vi "2_Analog_Meter_Reader(Training).vi"() -> ()   [LabVIEW 2020]
doc: "This example demonstrating the usage of Deep Learning toolkit for solving geometrical objects recognition problem based on Multilayer perceptron (MLP) and Convolutional Neural Network (CNN)."
uses:
  <vilib>/Ngene/DeepLTK/Toolkit/NN_Train/Controls/NN_LR_Policy_Cfg.ctl
  <vilib>/Ngene/DeepLTK/Toolkit/NN_Train/Controls/NN_LR_Policy_Type.ctl
  <vilib>/Ngene/DeepLTK/Toolkit/NN_Train/Controls/NN_Train_Params.ctl
  <vilib>/Ngene/DeepLTK/Toolkit/NN_Train/Controls/NN_Train_Optimizer.ctl
  <vilib>/Ngene/DeepLTK/Toolkit/NN_Train/Controls/NN_Train_Data_Sampling.ctl
  Controls/Regression_Report.ctl
  <vilib>/Ngene/DeepLTK/Toolkit/NN_Layers/Layers/FC/Controls/NN_Layer_Config(FC).ctl
  <vilib>/Ngene/DeepLTK/Toolkit/NN_Activations/Controls/NN_Activation_Type.ctl
  <vilib>/Ngene/DeepLTK/Toolkit/NN_Layers/Controls/NN_Layer_Init_Params.ctl
  <vilib>/Ngene/DeepLTK/Toolkit/NN_Layers/Controls/NN_Layer_Weight_Init_Type.ctl
  <vilib>/Ngene/DeepLTK/Toolkit/NN_Layers/Layers/Input/Controls/NN_Layer_Config(Input3D).ctl
  <vilib>/Ngene/DeepLTK/Toolkit/NN_Data/Controls/NN_Dims(C,H,W).ctl
  <vilib>/Ngene/DeepLTK/Toolkit/NN_Network/Controls/NN_Save_Before_Destroy_Options.ctl
  <vilib>/Ngene/DeepLTK/Toolkit/NN_Layers/Layers/Conv2D/Controls/NN_Layer_Config(Conv2D).ctl
  <vilib>/Ngene/DeepLTK/Toolkit/NN_Layers/Layers/Conv2D/Controls/NN_Layer_Params(Conv2D).ctl
  <vilib>/Ngene/DeepLTK/Toolkit/NN_Layers/Layers/Conv2D/Controls/NN_Conv2D_Padding_Type.ctl
  <vilib>/Ngene/DeepLTK/Toolkit/NN_Layers/Layers/DropOut3D/Controls/NN_Layer_Config(DropOut3D).ctl
  cd255efe-81e1-4e35-9bfd-5e2bf705b7ac.vi
  <vilib>/Ngene/DeepLTK/Toolkit/NN_Layers/Layers/Input/NN_Layer_Create(Input3D).vi
  <vilib>/Ngene/DeepLTK/Toolkit/NN_Layers/Layers/Conv2D/NN_Layer_Create(Conv2D).vi
  <vilib>/Ngene/DeepLTK/Toolkit/NN_Layers/Layers/DropOut3D/NN_Layer_Create(DropOut3D).vi
  <vilib>/Ngene/DeepLTK/Toolkit/NN_Layers/Layers/FC/NN_Layer_Create(FC).vi
  <vilib>/Ngene/DeepLTK/Toolkit/NN_Train/Loss_Functions/NN_Set_Loss(MSE).vi
  <vilib>/ptbypt/Filters.llb/FIR Filter PtByPt.vi
  <vilib>/Ngene/DeepLTK/Toolkit/NN_Network/subVIs/NN_Predict/NN_Predict(In3D_Out1D).vi
  <vilib>/Ngene/DeepLTK/Toolkit/NN_Train/Eval_Loss/NN_Eval_Test_Error_Loss/NN_Eval(In3D_Out1D).vi
  <vilib>/Ngene/DeepLTK/Toolkit/NN_Data/subVIs/Dataset_Destroy/NN_Datasets_All_Destroy(In3D_Out1D).vi
  <vilib>/Ngene/DeepLTK/Toolkit/Deep_Learning_Toolkit_by_Ngene.lvlib
panel:
  in  "NN Device":enum16{"CPU", "GPU"}(ring)=enum."GPU"
  out "Train Speed (img/s)":dbl=1665.0883017080685 format="%#_3p"
  out "Train Speed (sec/batch)":dbl=0.07687280000027386 format="%#_3p"
  out "Elapsed Time":dbl=38.292933199998515 format="%<%H:%M:%S>t"
  out "Test.Dataset_Size":i32=200
  out "Train.Dataset_Size":i32=1000
  out "Loss Values":cluster{"Train_Loss":dbl, "Test_Loss":dbl}={"Train_Loss"=19.829761505126953, "Test_Loss"=0.26563704013824463} {"Test_Loss" format="%#_4g"}
  out "Session Data":T1={"Epochs"=60.03200149536133, "Tot_Iter"=469.0, "LR"=0.625, "LR_iter"=470.0} {"LR" format="%#_3g"}
  out "Loss Charts":cluster{"Filtered x":sgl, "Test_Loss":sgl}(graph)={"Filtered x"=19.829762, "Test_Loss"=0.26563704}
  in  "Image Folder(Test)":path=path "D:/DeepLTK_Examples/Analog_Meter/Test/Images"
  in  "Labels (Test)":path=path "D:/DeepLTK_Examples/Analog_Meter/Test/Labels.csv"
  in  "Stop":bool
  out "Regression Metrics":T2={"Graphs"=[{"Best Linear Fit"=[0.0, 0.7035179734230042, 1.407034993171692, 2.110553026199341, 2.814069986343384, 3.517587900161743, 4.221106052398682, 4.924623012542725, 5.628140926361084, 6.331657886505127, 7.035175800323486, 7.7386932373046875, 8.442211151123047, 9.145729064941406, 9.84924602508545, 10.552763938903809, 11.256280899047852, 11.959798812866211, 12.66331672668457, 13.366833686828613, 14.070351600646973, 14.773868560791016, 15.477387428283691, 16.180904388427734, 16.884422302246094, 17.587940216064453, 18.29145622253418, 18.99497413635254, 19.6984920501709, 20.402009963989258, 21.105527877807617, 21.809045791625977, 22.512563705444336, 23.216079711914062, 23.919597625732422, 24.62311553955078, 25.32663345336914, 26.0301513671875, 26.733667373657227, 27.437185287475586, 28.140703201293945, 28.844221115112305, 29.547739028930664, 30.251256942749023, 30.954774856567383, 31.65829086303711, 32.36180877685547, 33.06532669067383, 33.76884460449219, 34.47236251831055, 35.175880432128906, 35.879398345947266, 36.582916259765625, 37.28643035888672, 37.98994827270508, 38.69346618652344, 39.3969841003418, 40.100502014160156, 40.804019927978516, 41.507537841796875, 42.211055755615234, 42.914573669433594, 43.61809158325195, 44.32160949707031, 45.02512741088867, 45.728641510009766, 46.432159423828125, 47.135677337646484, 47.839195251464844, 48.5427131652832, 49.24623107910156, 49.94974899291992, 50.65326690673828, 51.35678482055664, 52.060302734375, 52.76382064819336, 53.46733856201172, 54.17085266113281, 54.87437057495117, 55.57788848876953, 56.28140640258789, 56.98492431640625, 57.68844223022461, 58.39196014404297, 59.09547805786133, 59.79899597167969, 60.50251388549805, 61.206031799316406, 61.909549713134766, 62.61306381225586, 63.31658172607422, 64.02010345458984, 64.72361755371094, 65.42713928222656, 66.13065338134766, 66.83416748046875, 67.53768920898438, 68.24120330810547, 68.9447250366211, 69.64823913574219, 70.35176086425781, 71.0552749633789, 71.75879669189453, 72.46231079101562, 73.16583251953125, 73.86934661865234, 74.57286071777344, 75.27638244628906, 75.97989654541016, 76.68341827392578, 77.38693237304688, 78.0904541015625, 78.7939682006836, 79.49748992919922, 80.20100402832031, 80.90452575683594, 81.60803985595703, 82.31156158447266, 83.01507568359375, 83.71858978271484, 84.42211151123047, 85.12562561035156, 85.82914733886719, 86.53266143798828, 87.2361831665039, 87.939697265625, 88.64321899414062, 89.34673309326172, 90.05024719238281, 90.75376892089844, 91.45728302001953, 92.16080474853516, 92.86431884765625, 93.56784057617188, 94.27135467529297, 94.9748764038086, 95.67839050292969, 96.38191223144531, 97.0854263305664, 97.78894805908203, 98.49246215820312, 99.19597625732422, 99.89949798583984, 100.60301208496094, 101.30653381347656, 102.01004791259766, 102.71356964111328, 103.41708374023438, 104.12060546875, 104.8241195678711, 105.52764129638672, 106.23115539550781, 106.9346694946289, 107.63819122314453, 108.34170532226562, 109.04522705078125, 109.74874114990234, 110.45226287841797, 111.15577697753906, 111.85929870605469, 112.56281280517578, 113.2663345336914, 113.9698486328125, 114.67337036132812, 115.37688446044922, 116.08039855957031, 116.78392028808594, 117.48743438720703, 118.19095611572266, 118.89447021484375, 119.59799194335938, 120.30150604248047, 121.0050277709961, 121.70854187011719, 122.41206359863281, 123.1155776977539, 123.819091796875, 124.52261352539062, 125.22612762451172, 125.92964935302734, 126.63316345214844, 127.33668518066406, 128.0402069091797, 128.74371337890625, 129.44723510742188, 130.1507568359375, 130.85427856445312, 131.5577850341797, 132.2613067626953, 132.96482849121094, 133.6683349609375, 134.37185668945312, 135.07537841796875, 135.77890014648438, 136.48240661621094, 137.18592834472656, 137.8894500732422, 138.5929718017578, 139.29647827148438, 140.0], "Array 3"=[1.2962517, 0.8418449, 2.5273826, 2.343565, 2.8205507, 3.8072836, 4.6100063, 5.491647, 5.592317, 6.4402056, 7.130179, 7.626676, 8.663867, 9.402606, 10.082472, 10.911277, 11.306467, 11.893557, 12.946919, 13.433682, 14.082973, 14.6786, 15.393217, 16.218815, 16.990051, 17.676376, 18.30693, 19.016312, 19.612173, 20.773912, 21.31578, 22.13029, 22.531034, 23.691423, 23.968306, 24.432058, 25.35231, 25.968063, 26.499355, 27.619349, 28.226751, 28.762365, 29.584696, 30.380968, 30.965748, 31.767052, 32.254795, 32.90442, 33.4425, 33.98359, 35.325848, 36.042965, 36.61501, 37.261543, 37.82164, 38.58534, 39.109116, 39.722027, 40.41493, 40.994183, 41.832478, 42.44226, 43.27765, 44.356384, 44.996952, 45.652363, 46.350983, 46.879814, 47.487907, 48.07724, 48.716225, 49.195232, 50.24242, 51.0404, 51.87234, 52.24179, 52.91254, 53.425343, 54.369644, 55.455452, 56.149426, 56.705288, 57.2974, 57.85313, 58.777023, 59.593285, 60.04869, 60.95353, 61.77137, 62.53276, 63.122807, 63.74631, 64.20286, 65.17948, 65.843544, 66.83675, 67.39386, 68.15095, 68.68514, 69.15952, 69.499016, 70.364685, 71.12549, 72.3465, 72.72487, 73.790794, 74.30419, 74.74704, 75.398346, 76.282745, 77.012344, 77.77125, 78.58103, 79.15686, 79.749214, 80.42085, 81.20427, 81.76548, 82.57208, 83.061516, 83.735374, 84.47109, 85.10138, 85.91469, 86.56425, 87.1886, 88.19484, 88.94755, 89.88243, 90.78077, 91.201805, 92.01801, 92.4638, 92.76064, 93.48943, 94.34645, 95.05727, 95.58946, 96.37274, 96.85058, 97.76942, 98.29599, 99.13515, 99.81821, 100.50452, 101.524635, 102.11071, 102.60852, 103.29312, 103.88792, 104.80595, 105.36168, 106.023285, 106.71556, 107.36465, 108.053665, 108.94084, 109.85283, 110.555466, 111.16668, 111.92209, 113.046684, 113.679955, 114.0655, 115.12781, 115.78996, 116.65573, 116.89387, 117.78699, 118.39015, 119.00426, 120.01063, 120.73522, 121.56977, 122.11879, 122.91684, 123.60596, 124.266556, 125.044495, 125.64256, 126.34403, 126.98127, 127.77769, 128.66357, 128.89668, 129.37943, 130.17139, 130.81459, 131.21861, 132.22198, 133.08286, 133.59778, 134.10455, 134.84381, 135.72055, 137.03716, 137.40094, 137.66003, 137.51796, 138.29012]}, {"Best Linear Fit"=[1.1465655086328974, 0.6890048561897085, 2.3862414129443907, 2.201147959522832, 2.6814442810750747, 3.6750258871861514, 4.48332006058631, 5.371079722444516, 5.472448785683747, 6.326222219723485, 7.020984492338908, 7.520927698919899, 8.56531747444022, 9.309183875628419, 9.993768477460348, 10.828325958184701, 11.226259105607417, 11.817423473743009, 12.87809742648757, 13.368238917194887, 14.022035548748985, 14.621797424694607, 15.341374161798484, 16.17270217544307, 16.949291538335128, 17.640380208121634, 18.275310913345354, 18.98961563907013, 19.589612786926114, 20.759415454631, 21.305044625029957, 22.125206345720784, 22.52873320284901, 23.697176094941362, 23.97598003077316, 24.442951559630774, 25.369590624896187, 25.989617574818702, 26.524597090173177, 27.652363869697975, 28.26398248963226, 28.803314055181648, 29.631352103255235, 30.433151091415798, 31.021989628666113, 31.828855125394277, 32.319983797831604, 32.974116532114785, 33.51593333727239, 34.0607769875788, 35.412351693521735, 36.13444632021322, 36.71046109790862, 37.361482481213976, 37.9254667017951, 38.69446590477087, 39.22187830725335, 39.83904358251107, 40.53675443635409, 41.12002903299775, 41.96414239445679, 42.57815790699621, 43.419344293831664, 44.505566855454354, 45.150580642550665, 45.8105404378627, 46.514009211601724, 47.04651116969608, 47.65882504213281, 48.252248020607865, 48.8956677204748, 49.37800010434517, 50.43245615660163, 51.23597599073511, 52.07368995623235, 52.44570382148143, 53.12110897763525, 53.63747032238536, 54.588326069428206, 55.681670167733486, 56.38046039148363, 56.94018090887292, 57.536404103228016, 58.095990179525664, 59.02629564541866, 59.848222385583945, 60.306789425627365, 61.21790822715708, 62.0414252133777, 62.80810050605522, 63.402241784077006, 64.03007399966242, 64.48978955074581, 65.47319156548636, 66.14186314353631, 67.14195890068385, 67.70293932316045, 68.46528177151329, 69.0031844203173, 69.48085746006902, 69.82270658552935, 70.69438421194752, 71.46046796382186, 72.68995095269035, 73.07094932403467, 74.14427322320853, 74.66123379110992, 75.1071556861916, 75.76298237822938, 76.65352016921686, 77.38818311738916, 78.15235396458823, 78.96775839122222, 79.54758361357194, 80.14404880189198, 80.82034895159869, 81.60920318322187, 82.17430902662463, 82.98650991410366, 83.47934022664367, 84.15787593964555, 84.89870013098877, 85.53336195402922, 86.35231562548235, 87.00638305980674, 87.63506801603052, 88.64829290606968, 89.4062256866169, 90.34759757493845, 91.25217101589257, 91.67612907777522, 92.49800204150384, 92.94688164060149, 93.24578644021967, 93.97963505949407, 94.84260090317433, 95.55834991034067, 96.0942397839442, 96.8829557333017, 97.36410887673973, 98.28932478702085, 98.81955277007955, 99.66453423687315, 100.35233486167569, 101.043408166766, 102.07060724798706, 102.66074986382623, 103.1620153945728, 103.85136785369019, 104.45029139340012, 105.37469297478334, 105.93428289225504, 106.6004807542189, 107.29756165551828, 107.95115278426087, 108.64495332292435, 109.53828748861784, 110.45660465031106, 111.16411818032128, 111.77957413312821, 112.5402264649005, 113.67262762091265, 114.31029324205761, 114.69851302060974, 115.76819548678732, 116.43494647781392, 117.30672397475732, 117.54651310579675, 118.445831820655, 119.05318289622339, 119.67155045895774, 120.68490594891448, 121.4145292767375, 122.25487060528268, 122.80770005643218, 123.6112890316985, 124.3051894408872, 124.97037323290274, 125.75371153859486, 126.35593080563686, 127.06226893638878, 127.70392937854231, 128.50587433131665, 129.39791018018235, 129.63263664382822, 130.11872953709033, 130.91618799857812, 131.5638560369407, 131.97068246257504, 132.98101878973108, 133.8478642191985, 134.36636125671856, 134.8766535464749, 135.62104234733346, 136.50386706083515, 137.829609871314, 138.19591959310375, 138.45681213435577, 138.3137514481604, 139.0912665339977], "Array 3"=[1.2962517, 0.8418449, 2.5273826, 2.343565, 2.8205507, 3.8072836, 4.6100063, 5.491647, 5.592317, 6.4402056, 7.130179, 7.626676, 8.663867, 9.402606, 10.082472, 10.911277, 11.306467, 11.893557, 12.946919, 13.433682, 14.082973, 14.6786, 15.393217, 16.218815, 16.990051, 17.676376, 18.30693, 19.016312, 19.612173, 20.773912, 21.31578, 22.13029, 22.531034, 23.691423, 23.968306, 24.432058, 25.35231, 25.968063, 26.499355, 27.619349, 28.226751, 28.762365, 29.584696, 30.380968, 30.965748, 31.767052, 32.254795, 32.90442, 33.4425, 33.98359, 35.325848, 36.042965, 36.61501, 37.261543, 37.82164, 38.58534, 39.109116, 39.722027, 40.41493, 40.994183, 41.832478, 42.44226, 43.27765, 44.356384, 44.996952, 45.652363, 46.350983, 46.879814, 47.487907, 48.07724, 48.716225, 49.195232, 50.24242, 51.0404, 51.87234, 52.24179, 52.91254, 53.425343, 54.369644, 55.455452, 56.149426, 56.705288, 57.2974, 57.85313, 58.777023, 59.593285, 60.04869, 60.95353, 61.77137, 62.53276, 63.122807, 63.74631, 64.20286, 65.17948, 65.843544, 66.83675, 67.39386, 68.15095, 68.68514, 69.15952, 69.499016, 70.364685, 71.12549, 72.3465, 72.72487, 73.790794, 74.30419, 74.74704, 75.398346, 76.282745, 77.012344, 77.77125, 78.58103, 79.15686, 79.749214, 80.42085, 81.20427, 81.76548, 82.57208, 83.061516, 83.735374, 84.47109, 85.10138, 85.91469, 86.56425, 87.1886, 88.19484, 88.94755, 89.88243, 90.78077, 91.201805, 92.01801, 92.4638, 92.76064, 93.48943, 94.34645, 95.05727, 95.58946, 96.37274, 96.85058, 97.76942, 98.29599, 99.13515, 99.81821, 100.50452, 101.524635, 102.11071, 102.60852, 103.29312, 103.88792, 104.80595, 105.36168, 106.023285, 106.71556, 107.36465, 108.053665, 108.94084, 109.85283, 110.555466, 111.16668, 111.92209, 113.046684, 113.679955, 114.0655, 115.12781, 115.78996, 116.65573, 116.89387, 117.78699, 118.39015, 119.00426, 120.01063, 120.73522, 121.56977, 122.11879, 122.91684, 123.60596, 124.266556, 125.044495, 125.64256, 126.34403, 126.98127, 127.77769, 128.66357, 128.89668, 129.37943, 130.17139, 130.81459, 131.21861, 132.22198, 133.08286, 133.59778, 134.10455, 134.84381, 135.72055, 137.03716, 137.40094, 137.66003, 137.51796, 138.29012]}, {"Best Linear Fit"=[0.0, 140.0], "Array 3"=[0.0, 140.0]}], "y=k*x+b"="y = 0.993*x + 0.158", "R"=0.9999755, "R^2"=0.999951, "MAE"=0.40923384, "MSE"=0.26563704} {"R" format="%#_7g"}
  in  "Evaluate Model":bool
  in  "LR Update Policy":T3={"Policy_Type"=enum."Step", "LR0"=20.0, "k"=10.0, "WarmUp_Policy"=enum."Ramp", "WarmUp_Iter"=50, "WarmUp_Ratio"=50.0} {"WarmUp_Ratio" min=1; "WarmUp_Iter" min=1; "LR0" format="%.7f"}
  in  "Train_Params":T5={"Optimizer"=enum."Adam", "Beta_1"=0.9, "Beta_2"=0.999, "Weight Decay(L1)"=3e-09, "Weight Decay(L2)"=3e-09, "Data_Sampling"=enum."Random"}
  in  "Image Folder(Train)":path=path "D:/DeepLTK_Examples/Analog_Meter/Train/Images"
  in  "Labels (Train)":path=path "D:/DeepLTK_Examples/Analog_Meter/Train/Labels.csv"
  in  "Max_Epochs_to_Train":sgl=60.0
  in  "Input Height":i32=256
  in  "Input Width":i32=256
  out "Test_Loss":sgl=0.26563704
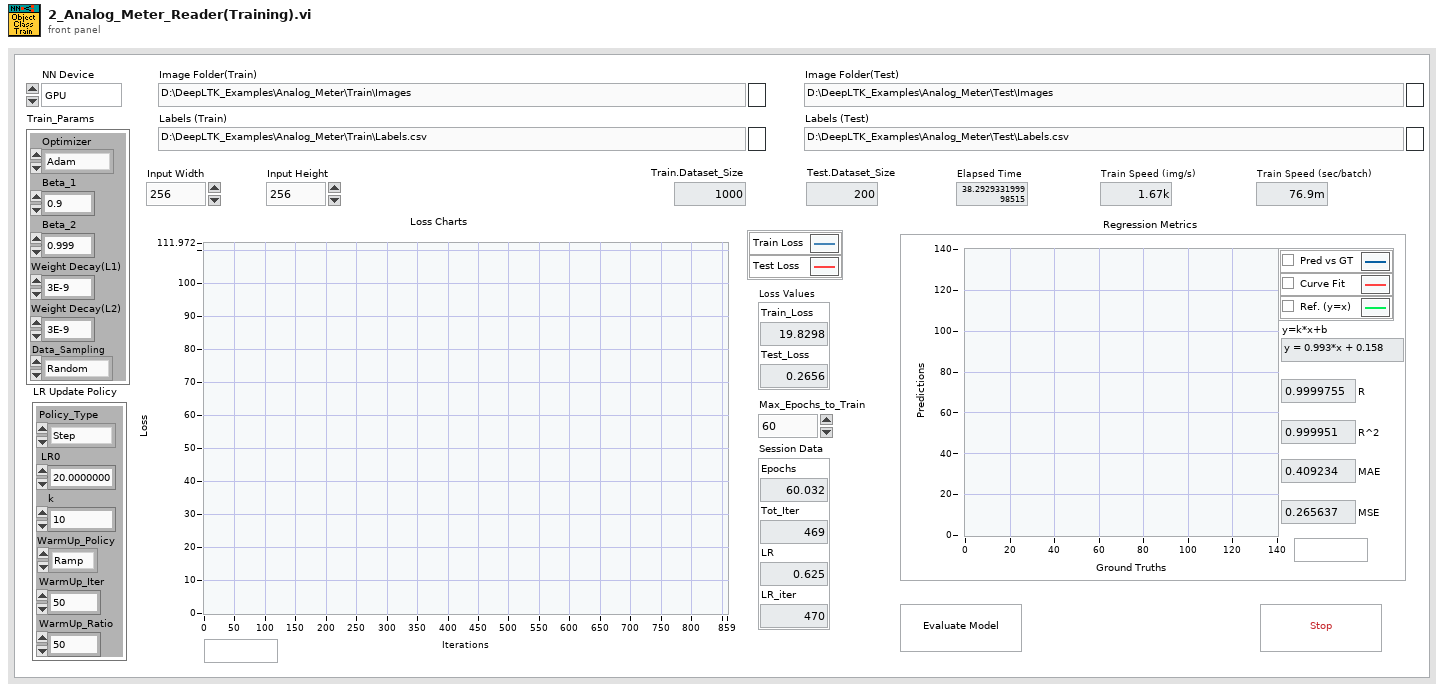
[diagram p1: front panel]
types:
  T1 = cluster{"Epochs":dbl, "Tot_Iter":dbl, "LR":dbl, "LR_iter":dbl}
  T2 = typedef "Regression_Report.ctl" = cluster{"Graphs":cluster{"Best Linear Fit":dbl[], "Array 3":sgl[]}[], "y=k*x+b":string, "R":sgl, "R^2":sgl, "MAE":sgl, "MSE":sgl}
  T3 = typedef "Deep_Learning_Toolkit_by_Ngene.lvlib/NN_LR_Policy_Cfg.ctl" = cluster{"Policy_Type":T4, "LR0":dbl, "k":sgl, "WarmUp_Policy":enum16{"Step", "Ramp"}, "WarmUp_Iter":i32, "WarmUp_Ratio":sgl}
  T4 = typedef "Deep_Learning_Toolkit_by_Ngene.lvlib/NN_LR_Policy_Type.ctl" = enum16{"Manual", "Step", "Exp", "1/t"}
  T5 = typedef "Deep_Learning_Toolkit_by_Ngene.lvlib/NN_Train_Params.ctl" = cluster{"Optimizer":T6, "Beta_1":sgl, "Beta_2":sgl, "Weight Decay(L1)":sgl, "Weight Decay(L2)":sgl, "Data_Sampling":T7}
  T6 = typedef "Deep_Learning_Toolkit_by_Ngene.lvlib/NN_Train_Optimizer.ctl" = enum16{"SGD", "Adam", "Adagrad", "Adadelta", "RMSProp", "Nesterov"}
  T7 = typedef "Deep_Learning_Toolkit_by_Ngene.lvlib/NN_Train_Data_Sampling.ctl" = enum16{"Random", "Sequential"}
  T8 = typedef "Deep_Learning_Toolkit_by_Ngene.lvlib/NN_Layer_Config(DropOut3D).ctl" = cluster{"Name":string, "Probability":sgl}
  T9 = typedef "Deep_Learning_Toolkit_by_Ngene.lvlib/NN_Layer_Config(FC).ctl" = cluster{"Name":string, "Size":i32, "BN":bool, "Activation":T10, "Init_Params":T11, "Custom_Params":string}
  T10 = typedef "Deep_Learning_Toolkit_by_Ngene.lvlib/NN_Activation_Type.ctl" = enum16{"Sigmoid", "ReLU", "LReLU", "ReLU6", "tanh", "Swish", "Mish", "None"}
  T11 = typedef "Deep_Learning_Toolkit_by_Ngene.lvlib/NN_Layer_Init_Params.ctl" = cluster{"Init_Type":T12, "Value":sgl}
  T12 = typedef "Deep_Learning_Toolkit_by_Ngene.lvlib/NN_Layer_Weight_Init_Type.ctl" = enum16{"Const", "Uniform", "Gaussian", "Xavier"}
  T13 = typedef "Deep_Learning_Toolkit_by_Ngene.lvlib/NN_Layer_Config(Conv2D).ctl" = cluster{"Name":string, "Conv_Params":T14, "BN?":bool, "Activation":T10, "Init_Params":T11, "Custom_Params":string}
  T14 = typedef "Deep_Learning_Toolkit_by_Ngene.lvlib/NN_Layer_Params(Conv2D).ctl" = cluster{"Filters":i32, "Kernel_Size":i32, "Stride":i32, "Pad_Type":T15, "Pad_Size":i32}
  T15 = typedef "Deep_Learning_Toolkit_by_Ngene.lvlib/NN_Conv2D_Padding_Type.ctl" = enum16{"Pad_Size", "Valid", "Same"}
  T16 = typedef "Deep_Learning_Toolkit_by_Ngene.lvlib/NN_Save_Before_Destroy_Options.ctl" = cluster{"CFG?":bool, "Weights?":bool, "Render?":bool}
  T17 = typedef "Deep_Learning_Toolkit_by_Ngene.lvlib/NN_Layer_Config(Input3D).ctl" = cluster{"Name":string, "Dims":T18}
  T18 = typedef "Deep_Learning_Toolkit_by_Ngene.lvlib/NN_Dims(C,H,W).ctl" = cluster{"C":i32, "H":i32, "W":i32}
  T19 = typedef "Deep_Learning_Toolkit_by_Ngene.lvlib/NN_DataSets_All(In3D_Out1D).ctl" = cluster{"Train":T20, "Validation":T20, "Test":T20}
  T20 = typedef "Deep_Learning_Toolkit_by_Ngene.lvlib/NN_DataSet(In3D_Out1D).ctl" = cluster{"Inputs Ref.":T21, "Outputs Ref.":T22, "Dataset_Size":i32, "Outputs_idx Ref.":T23, "Dims_In":T18, "Dims_Out":i32, "Labels":string[], "File Paths":path[]}
  T21 = typedef "Deep_Learning_Toolkit_by_Ngene.lvlib/NN_Data_ref(4D_SGL).ctl" = refnum<data-value>
  T22 = typedef "Deep_Learning_Toolkit_by_Ngene.lvlib/NN_Data_ref(2D_SGL).ctl" = refnum<data-value>
  T23 = typedef "Deep_Learning_Toolkit_by_Ngene.lvlib/NN_Data_ref(1D_I32).ctl" = refnum<data-value>
  T24 = typedef "Deep_Learning_Toolkit_by_Ngene.lvlib/NN.ctl" = cluster{"Name":string, "No of Layers":i32, "mBatch":i32, "Layers":T25[], "Dimty":T26, "Dims_In":T18, "Dims_Out":T18, "Working_Dir":path, "Train?":bool, "Train_Params":T5, "LR_Update_Policy":T3, "Session Data":T27, "Ground_truth":T28, "NNg_hdls":T29, "NN_Device":T30, "GPU Id":i32, "Labels":string[], "Receptive Field":T31[], "Loss_Type":T32, "Loss_Cfg_Prms":variant}
  T25 = typedef "Deep_Learning_Toolkit_by_Ngene.lvlib/NN_Layer_ref.ctl" = refnum<data-value>
  T26 = typedef "Deep_Learning_Toolkit_by_Ngene.lvlib/NN_In_Out_Dim-ty.ctl" = enum8{"In1D_Out1D", "In3D_Out1D", "In3D_Out3D", "In3D_OutBBox"}
  T27 = typedef "Deep_Learning_Toolkit_by_Ngene.lvlib/NN_Train_Session_Data.ctl" = cluster{"Epochs":sgl, "Tot_Iter":i32, "LR":sgl, "LR_iter":i32}
  T28 = typedef "Deep_Learning_Toolkit_by_Ngene.lvlib/NN_Ground_truth.ctl" = cluster{"Y":variant, "Y_idx":T23}
  T29 = typedef "Deep_Learning_Toolkit_by_Ngene.lvlib/nng_cuda_handles.ctl" = cluster{"cudnn":u64, "cublas":u64, "stream":u64, "curand":u64}
  T30 = typedef "Deep_Learning_Toolkit_by_Ngene.lvlib/NN_Device.ctl" = enum16{"CPU", "GPU"}
  T31 = typedef "Deep_Learning_Toolkit_by_Ngene.lvlib/NN_Dims(V,H).ctl" = cluster{"V":i32, "H":i32}
  T32 = typedef "Deep_Learning_Toolkit_by_Ngene.lvlib/NN_Loss_Type.ctl" = enum16{"None", "MSE", "CrossEntropy", "YOLO_v2"}
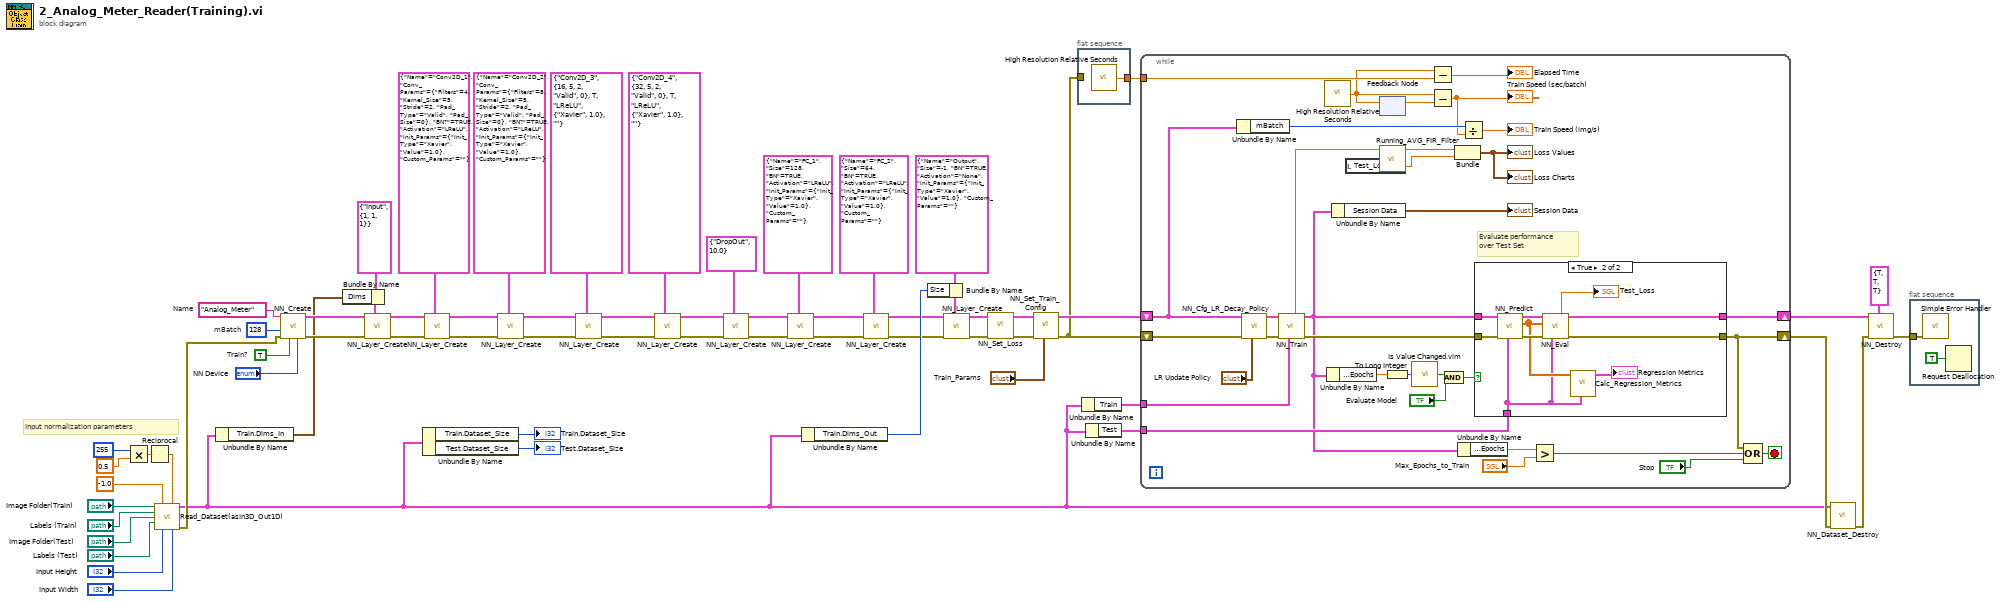
[diagram p0: block diagram]
diagram:
  w47 = TRUE  # Train?
  w59 = 128  # mBatch
  w64 = "Analog_Meter"  # Name
  # "Input normalization parameters"
  n1 = Multiply(x=u16 255 ("Shift"), y=sgl 0.5 ("Scale")) -> (x*y=w20:sgl)
  n2 = Reciprocal(x=w20) -> (1/x=w19:sgl)
  n3 = call "Read_Dataset(asIn3D_Out1D).vi"("Image Folder Path(Train)"="Image Folder(Train)", "Norm. Shift"=sgl -1.0 ("Scale"), "Norm. Scale"=w19, "Label File Path(Train)"="Labels (Train)", "Image Folder Path(Test)"="Image Folder(Test)", "Label File Path(Test)"="Labels (Test)", "Img Heigth"="Input Height", "Img Width"="Input Width") -> ("Datasets"=w1:T19, "error out"=w65:errorcluster)  [unwired: 6 in]
  n4 = Unbundle By Name(w1) -> ("Train.Dims_In"=w42:T18)
  n5 = call <vilib>:"NN_Create.vi"("NN_Device"="NN Device", "Train? (false)"=w47, "error in (no error)"=w65, "mBatch (1)"=w59, "Name"=w64) -> ("error out"=w62:errorcluster, "NN out"=w63:T24)  [unwired: 5 in]
  n6 = Bundle By Name(cluster=T17 {"Name"="Input", "Dims"={"C"=1, "H"=1, "W"=1}} ("Cluster"), "Dims"=w42) -> (w50:T17)
  n7 = call-poly <vilib>:"NN_Layer_Create.vi"("Input3D_Cfg"=w50, "error in (no error)"=w62, "NN In"=w63) -> ("error out"=w56:errorcluster, "NN out"=w57:T24)  [unwired: 6 in, 1 out]
  n8 = Unbundle By Name(w1) -> ("Train.Dataset_Size"=→"Train.Dataset_Size":i32, "Test.Dataset_Size"=→"Test.Dataset_Size":i32)
  n9 = call-poly <vilib>:"NN_Layer_Create.vi"("Conv2D_Cfg"=T13 {"Name"="Conv2D_1", "Conv_Params"={"Filters"=4, "Kernel_Size"=5, "Stride"=2, "Pad_Type"=enum."Valid", "Pad_Size"=0}, "BN?"=TRUE, "Activation"=enum."LReLU", "Init_Params"={"Init_Type"=enum."Xavier", "Value"=1.0}, "Custom_Params"=""}, "error in (no error)"=w56, "NN in"=w57) -> ("error out"=w16:errorcluster, "NN out"=w15:T24)  [unwired: 6 in, 1 out]
  n10 = call-poly <vilib>:"NN_Layer_Create.vi"("Conv2D_Cfg"=T13 {"Name"="Conv2D_2", "Conv_Params"={"Filters"=8, "Kernel_Size"=5, "Stride"=2, "Pad_Type"=enum."Valid", "Pad_Size"=0}, "BN?"=TRUE, "Activation"=enum."LReLU", "Init_Params"={"Init_Type"=enum."Xavier", "Value"=1.0}, "Custom_Params"=""}, "error in (no error)"=w16, "NN in"=w15) -> ("error out"=w39:errorcluster, "NN out"=w40:T24)  [unwired: 6 in, 1 out]
  n11 = call-poly <vilib>:"NN_Layer_Create.vi"("Conv2D_Cfg"=T13 {"Name"="Conv2D_3", "Conv_Params"={"Filters"=16, "Kernel_Size"=5, "Stride"=2, "Pad_Type"=enum."Valid", "Pad_Size"=0}, "BN?"=TRUE, "Activation"=enum."LReLU", "Init_Params"={"Init_Type"=enum."Xavier", "Value"=1.0}, "Custom_Params"=""}, "error in (no error)"=w39, "NN in"=w40) -> ("error out"=w7:errorcluster, "NN out"=w8:T24)  [unwired: 6 in, 1 out]
  n12 = call-poly <vilib>:"NN_Layer_Create.vi"("Conv2D_Cfg"=T13 {"Name"="Conv2D_4", "Conv_Params"={"Filters"=32, "Kernel_Size"=5, "Stride"=2, "Pad_Type"=enum."Valid", "Pad_Size"=0}, "BN?"=TRUE, "Activation"=enum."LReLU", "Init_Params"={"Init_Type"=enum."Xavier", "Value"=1.0}, "Custom_Params"=""}, "error in (no error)"=w7, "NN in"=w8) -> ("error out"=w5:errorcluster, "NN out"=w6:T24)  [unwired: 6 in, 1 out]
  n13 = call-poly <vilib>:"NN_Layer_Create.vi"("DropOut3D_Cfg"=T8 {"Name"="DropOut", "Probability"=10.0}, "error in (no error)"=w5, "NN in"=w6) -> ("error out"=w3:errorcluster, "NN out"=w4:T24)  [unwired: 6 in, 1 out]
  n14 = call-poly <vilib>:"NN_Layer_Create.vi"("FC_Cfg"=T9 {"Name"="FC_1", "Size"=128, "BN"=TRUE, "Activation"=enum."LReLU", "Init_Params"={"Init_Type"=enum."Xavier", "Value"=1.0}, "Custom_Params"=""} ("Layer_Config_Params"), "error in (no error)"=w3, "NN in"=w4) -> ("error out"=w17:errorcluster, "NN out"=w18:T24)  [unwired: 6 in, 1 out]
  n15 = Unbundle By Name(w1) -> ("Train.Dims_Out"=w41:i32)
  n16 = call-poly <vilib>:"NN_Layer_Create.vi"("FC_Cfg"=T9 {"Name"="FC_2", "Size"=64, "BN"=TRUE, "Activation"=enum."LReLU", "Init_Params"={"Init_Type"=enum."Xavier", "Value"=1.0}, "Custom_Params"=""} ("Layer_Config_Params"), "error in (no error)"=w17, "NN in"=w18) -> ("error out"=w22:errorcluster, "NN out"=w23:T24)  [unwired: 6 in, 1 out]
  n17 = Bundle By Name(cluster=T9 {"Name"="Output", "Size"=-1, "BN"=TRUE, "Activation"=enum."None", "Init_Params"={"Init_Type"=enum."Xavier", "Value"=1.0}, "Custom_Params"=""} ("Layer_Config_Params"), "Size"=w41) -> (w51:T9)
  n18 = call-poly <vilib>:"NN_Layer_Create.vi"("FC_Cfg"=w51, "error in (no error)"=w22, "NN in"=w23) -> ("error out"=w54:errorcluster, "NN out"=w55:T24)  [unwired: 6 in, 1 out]
  n19 = call-poly <vilib>:"NN_Set_Loss.vi"("error in (no error)"=w54, "NN in"=w55) -> ("error out"=w34:errorcluster, "NN out"=w35:T24)  [unwired: 8 in]
  n20 = call <vilib>:"NN_Set_Train_Config.vi"("NN_Train_Params"="Train_Params", "error in (no error)"=w34, "NN in"=w35) -> ("error out"=w48:errorcluster, "NN out"=w49:T24)  [unwired: 7 in]
  n21 = flat-sequence {
    tunnel: [w66] -> w61
    tunnel: w48 -> [_]
    frame #0 {
      n22 = call <vilib>:"High Resolution Relative Seconds.vi"() -> ("relative seconds"=w66:dbl)
    }
  }
  n23 = Unbundle By Name(w1) -> ("Train"=w45:T20)
  n24 = Unbundle By Name(w1) -> ("Test"=w58:T20)
  n25 = while {
    shift-right: [w67] -> w33
    shift-left: w48 -> [w84]
    shift-right: [w68] -> w32
    shift-left: w49 -> [w85]
    tunnel: w61 -> [w91]
    tunnel: w45 -> [w76]
    tunnel: w58 -> [w87]
    stop <- w97 stop-if-true
    # "Evaluate performance \nover Test Set"
    n26 = Unbundle By Name(w85) -> ("mBatch"=w89:i32)
    n27 = call <vilib>:"NN_Cfg_LR_Decay_Policy.vi"("LR_Decay_Params"="LR Update Policy", "error in (no error)"=w84, "NN in"=w85) -> ("error out"=w92:errorcluster, "NN out"=w98:T24)  [unwired: 7 in]
    n28 = call <vilib>:"NN_Train.vi"("Train Dataset"=w76, "error in (no error)"=w92, "NN in"=w98) -> ("error out"=w88:errorcluster, "NN out"=w81:T24, "Loss"=w93:sgl)  [unwired: 5 in, 1 out]
    n29 = call <vilib>:"High Resolution Relative Seconds.vi"() -> ("relative seconds"=w90:dbl)
    n30 = Unbundle By Name(w81) -> ("Session Data.Epochs"=w80:sgl)
    n31 = Unbundle By Name(w81) -> ("Session Data"=→"Session Data":T27)
    n32 = local read "Test_Loss"() -> (w96:sgl)
    n33 = feedback #1() -> (w99:dbl)  [unwired: 1 in]
    n34 = feedback-in #1(w90) -> ()
    n35 = call <vilib>:"Running_AVG_FIR_Filter.vi"("Numeric"=w93) -> ("Filtered x"=w94:sgl)  [unwired: 10 in]
    n36 = To Long Integer(number=w80) -> (32bit integer=w79:i32)
    n37 = call "Is Value Changed.vim"("value"=w79) -> ("changed or first call?"=w77:bool)
    n38 = Subtract(x=w90, y=w91) -> (x-y=→"Elapsed Time":dbl)
    n39 = Subtract(x=w90, y=w99) -> (x-y=w71:dbl)
    "Train Speed (sec/batch)" <- w71
    n40 = And(x=w77, y="Evaluate Model") -> (x .and. y?=w78:bool)
    n41 = Bundle("Filtered x"=w94, "Test_Loss"=w96) -> (→"Loss Values" →"Loss Charts":cluster{"Filtered x":sgl, "Test_Loss":sgl})  [unwired: 1 in]
    n42 = Unbundle By Name(w81) -> ("Session Data.Epochs"=w82:sgl)
    n43 = Divide(x=w89, y=w71) -> (x/y=→"Train Speed (img/s)":dbl)
    n44 = case shown="True" w78 {
      tunnel: w81 -> [w100 w111]
      tunnel: w88 -> [w101 w106]
      tunnel: [w101 w108] -> w67
      tunnel: w87 -> [_ w102]
      tunnel: [w100 w109] -> w68
      frame False {
      }
      frame True {
        n45 = call-poly <vilib>:"NN_Predict.vi"("Dataset"=w102, "error in (no error)"=w106, "NN in"=w111) -> ("error out"=w105:errorcluster, "Predictions"=w104:sgl[][], "NN out"=w107:T24)  [unwired: 6 in]
        n46 = call-poly <vilib>:"NN_Eval.vi"("NN in"=w107, "Predictions"=w104, "error in (no error)"=w105, "Dataset"=w102) -> ("Loss"=→"Test_Loss":sgl, "NN out"=w109:T24, "error out"=w108:errorcluster)  [unwired: 7 in, 2 out]
        n47 = call "Calc_Regression_Metrics.vi"("Dataset"=w102, "Predictions"=w104) -> ("Metrics"=→"Regression Metrics":T2)  [unwired: 9 in]
      }
    }
    n48 = Greater?(x=w82, y="Max_Epochs_to_Train") -> (0:w74:bool)
    n49 = Compound Arithmetic op=OR(w67, w74, "Stop") -> (w97:bool)
  }
  n50 = call-poly <vilib>:"NN_Dataset_Destroy.vi"("error in (no error)"=w33, "Datasets_All(In3D_Out1D)"=w1) -> ("error out"=w31:errorcluster)  [unwired: 9 in]
  n51 = call <vilib>:"NN_Destroy.vi"("Save (T, T, T)"=T16 {"CFG?"=TRUE, "Weights?"=TRUE, "Render?"=TRUE} ("Save_Config"), "error in (no error)"=w31, "NN in"=w32) -> ("error out"=w43:errorcluster)  [unwired: 8 in]
  n52 = flat-sequence {
    tunnel: w43 -> [w113]
    frame #0 {
      n53 = call <vilib>:"Simple Error Handler.vi"("error in (no error)"=w113) -> ()  [unwired: 4 in, 5 out]
      n54 = Request Deallocation(TRUE ("flag")) -> ()
    }
  }
